vi "HEWH RLT Channel Test Labels.vi"(0 "LV Program":T3=enum."HEWH", 11 "Error In":errorcluster) -> (4 "Station A":T2, 6 "Station B":T2, 8 "Station C":T2, 10 "Station D":T2, 15 "Error Out":errorcluster)   [LabVIEW 2023]
uses:
  Type Definitions/HEWH Channel Label RLT.ctl
  Custom Instrument Control/MW100/Type Definitions/Station ID Selector.ctl
  Type Definitions/HEWH RLT Stations.ctl
  Type Definitions/HEWH Label Channel.ctl
  Utility/Save File/File Setup (Public)/Type Definition/Save File DOE LabView Program.ctl
  Type Definitions/HEWH Agilent Cluster.ctl
  Custom Instrument Control/MW100/Type Definitions/HEWH MW100 Channel Numbers.ctl
  Type Definitions/PRAT Channel Settings.ctl
  <vilib>/Utility/file.llb/Write Delimited Spreadsheet (string).vi
  <vilib>/Utility/file.llb/Read Delimited Spreadsheet (string).vi
  Utility/Save File/File Setup.lvlib
panel:
  out "Agilent Labels_Channels":T1[](array[typedef])
  in  "Tab Control":enum32{"Data Output", "Error"}(tab)
  out "Raw Data (Read)":string[][](array[string])
  out "Description":string="Thermocouple Setup"
  in  "Read":bool
  in  "Write":bool
  in  "Initialize":bool
  in  "Complete":bool
  in  "Panel 3":T4[][](array[typedef])=[[{"Label"="T3-1", "Unit"=enum.""}, {"Label"="T3-2", "Unit"=enum.""}, {"Label"="T3-3", "Unit"=enum.""}, {"Label"="T3-4", "Unit"=enum.""}, {"Label"="T3-5", "Unit"=enum.""}, {"Label"="T3-6", "Unit"=enum.""}], [{"Label"="T3-7", "Unit"=enum.""}, {"Label"="T3-8", "Unit"=enum.""}, {"Label"="T3-9", "Unit"=enum.""}, {"Label"="T3-10", "Unit"=enum.""}, {"Label"="T3-11", "Unit"=enum.""}, {"Label"="T3-12", "Unit"=enum.""}], [{"Label"="T3-13", "Unit"=enum.""}, {"Label"="T3-14", "Unit"=enum.""}, {"Label"="T3-15", "Unit"=enum.""}, {"Label"="T3-16", "Unit"=enum.""}, {"Label"="T3-17", "Unit"=enum.""}, {"Label"="T3-18", "Unit"=enum.""}]]
  in  "Panel 2":T4[][](array[typedef])=[[{"Label"="T2-1", "Unit"=enum.""}, {"Label"="T2-2", "Unit"=enum.""}, {"Label"="T2-3", "Unit"=enum.""}, {"Label"="T2-4", "Unit"=enum.""}, {"Label"="T2-5", "Unit"=enum.""}, {"Label"="T2-6", "Unit"=enum.""}], [{"Label"="T2-7", "Unit"=enum.""}, {"Label"="T2-8", "Unit"=enum.""}, {"Label"="T2-9", "Unit"=enum.""}, {"Label"="T2-10", "Unit"=enum.""}, {"Label"="T2-11", "Unit"=enum.""}, {"Label"="T2-12", "Unit"=enum.""}], [{"Label"="T2-13", "Unit"=enum.""}, {"Label"="T2-14", "Unit"=enum.""}, {"Label"="T2-15", "Unit"=enum.""}, {"Label"="T2-16", "Unit"=enum.""}, {"Label"="T2-17", "Unit"=enum.""}, {"Label"="T2-18", "Unit"=enum.""}]]
  in  "Panel 1":T4[][](array[typedef])=[[{"Label"="T1 - IN", "Unit"=enum."A"}, {"Label"="T1 - OUT", "Unit"=enum."A"}, {"Label"="T2 - IN", "Unit"=enum."B"}, {"Label"="T2 - OUT", "Unit"=enum."B"}, {"Label"="T3 - IN", "Unit"=enum."C"}, {"Label"="T3 - OUT", "Unit"=enum."C"}], [{"Label"="T4 - IN", "Unit"=enum."D"}, {"Label"="T4 - OUT", "Unit"=enum."D"}, {"Label"="T1-9", "Unit"=enum.""}, {"Label"="T1-10", "Unit"=enum.""}, {"Label"="T1-11", "Unit"=enum.""}, {"Label"="T1-12", "Unit"=enum.""}], [{"Label"="T1-13", "Unit"=enum.""}, {"Label"="T1-14", "Unit"=enum.""}, {"Label"="T1-15", "Unit"=enum.""}, {"Label"="T1-16", "Unit"=enum.""}, {"Label"="T1-17", "Unit"=enum.""}, {"Label"="T1-18", "Unit"=enum.""}]]
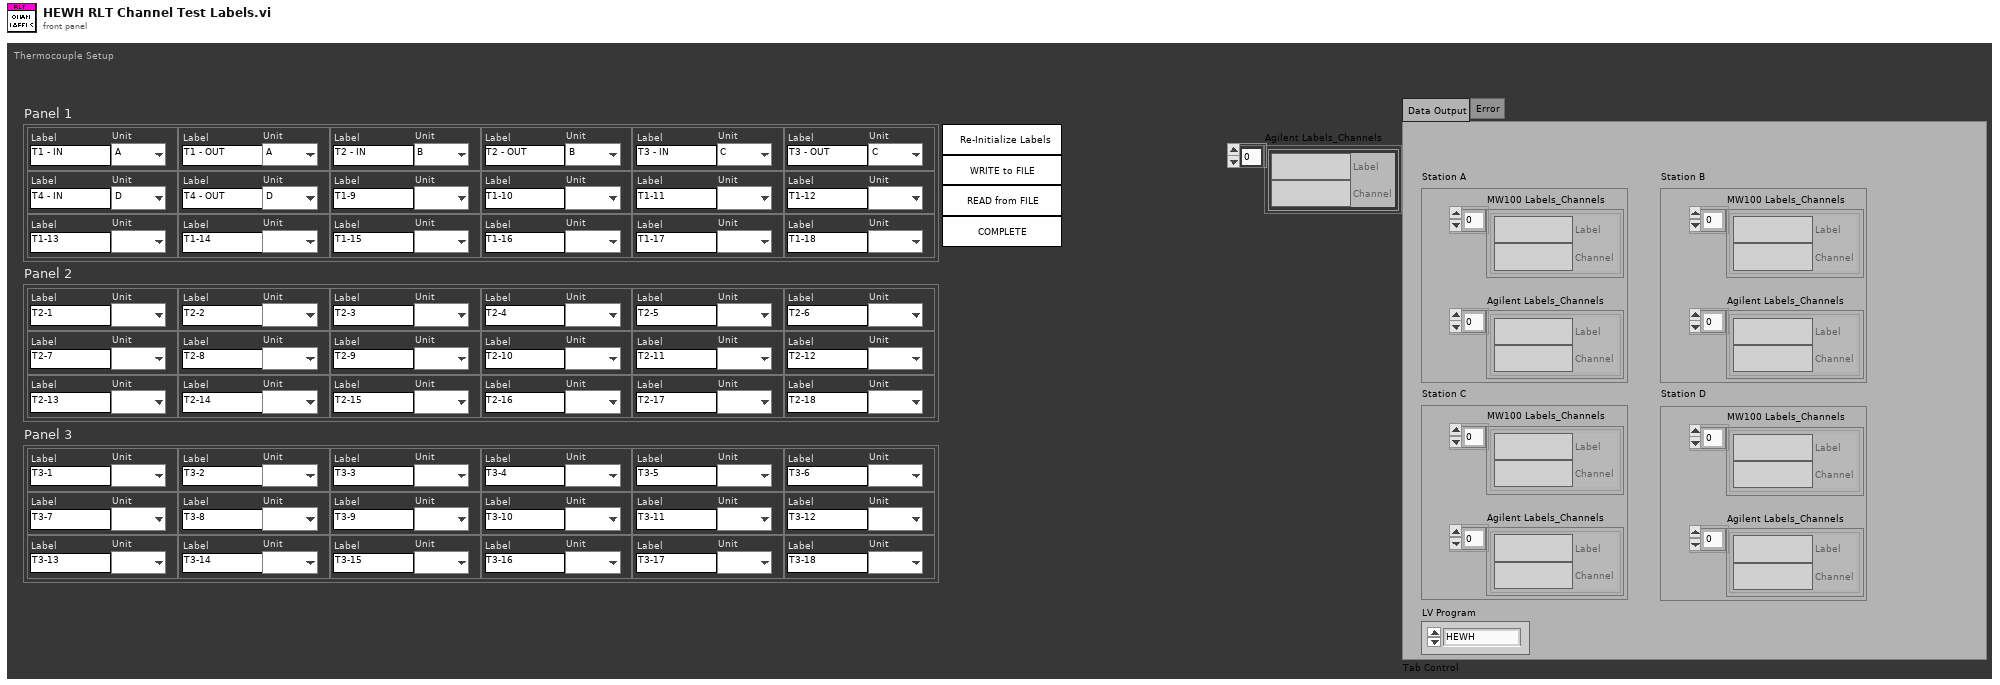
[diagram p1: front panel]
types:
  T1 = typedef "HEWH Label Channel.ctl" = cluster{"Label":string, "Channel":string}
  T2 = typedef "HEWH RLT Stations.ctl" = cluster{"MW100 Labels_Channels":T1[], "Agilent Labels_Channels":T1[]}
  T3 = typedef "File Setup.lvlib/Save File DOE LabView Program.ctl" = enum16{"No Name Found", "DOE Stand", "Dishwasher Kitchen", "Portable Stand", "HEWH", "Dryer", "Dryer WILT", "HCC", "PRAT", "HEWH RLT", "Refrigeration", "Gas Water Heater"}
  T4 = typedef "HEWH Channel Label RLT.ctl" = cluster{"Label":string, "Unit":T5}
  T5 = typedef "Station ID Selector.ctl" = enum16{"", "A", "B", "C", "D", "Global"}
  T6 = typedef "HEWH Agilent Cluster.ctl" = cluster{"Label":string, "Agilent Channel":string, "Panel ID":string, "Source":string, "Temperature":dbl}
  T7 = enum8{"Enabled", "Disabled", "Disabled and Grayed Out"}
  T8 = typedef "PRAT Channel Settings.ctl" = string
  T9 = typedef "HEWH MW100 Channel Numbers.ctl" = string
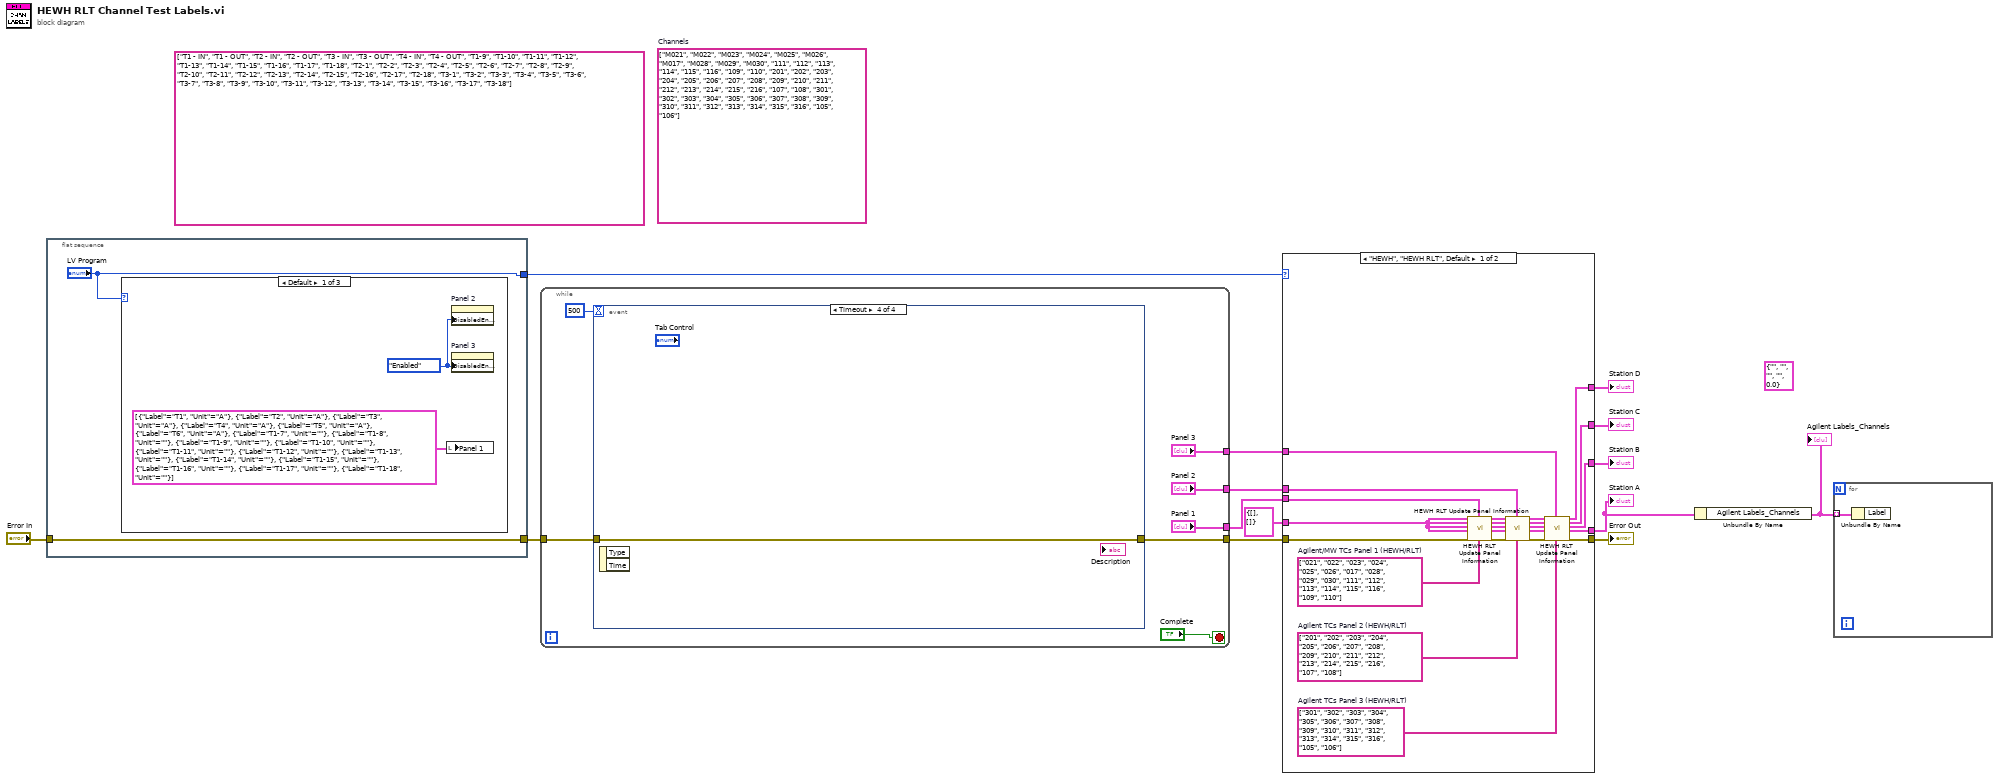
[diagram p0: block diagram]
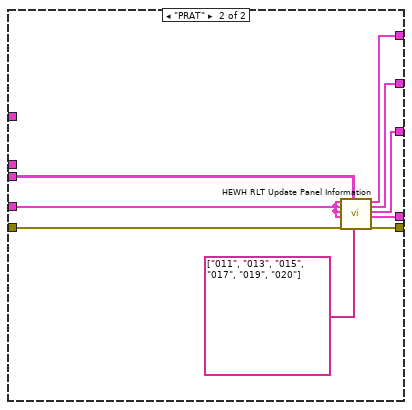
[diagram p2: hidden frame]
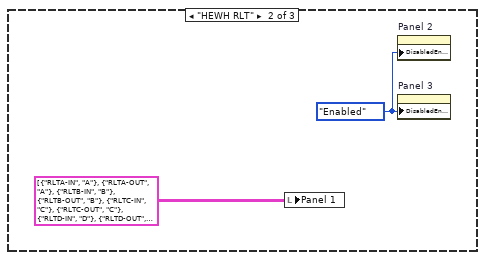
[diagram p3: hidden frame]
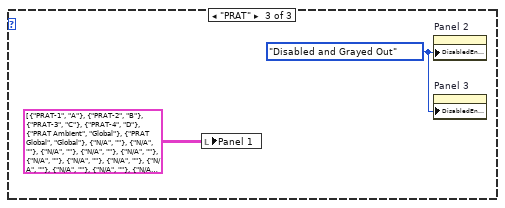
[diagram p4: hidden frame]
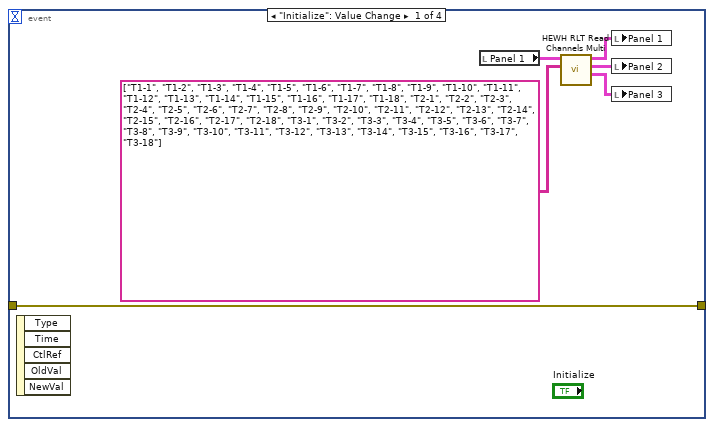
[diagram p5: hidden frame]
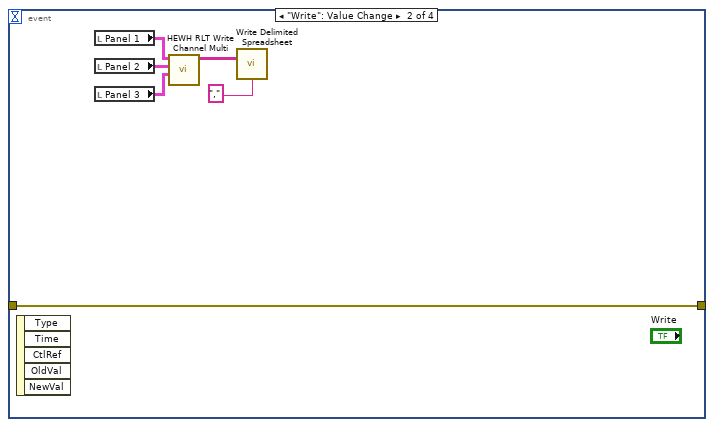
[diagram p6: hidden frame]
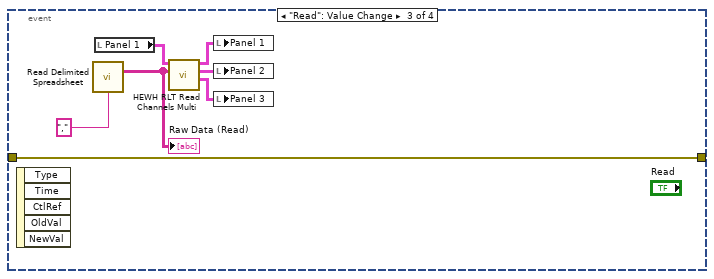
[diagram p7: hidden frame]
diagram:
  (unwired) T6 {"Label"="", "Agilent Channel"="", "Panel ID"="", "Source"="", "Temperature"=0.0} ("Agilent Cluster")
  (unwired) string[][] [["M021", "M022", "M023", "M024", "M025", "M026"], ["M017", "M028", "M029", "M030", "111", "112"], ["113", "114", "115", "116", "109", "110"], ["201", "202", "203", "204", "205", "206"], ["207", "208", "209", "210", "211", "212"], ["213", "214", "215", "216", "107", "108"], ["301", "302", "303", "304", "305", "306"], ["307", "308", "309", "310", "311", "312"], ["313", "314", "315", "316", "105", "106"]]  # Channels
  (unwired) string[][] [["T1 - IN", "T1 - OUT", "T2 - IN", "T2 - OUT", "T3 - IN", "T3 - OUT"], ["T4 - IN", "T4 - OUT", "T1-9", "T1-10", "T1-11", "T1-12"], ["T1-13", "T1-14", "T1-15", "T1-16", "T1-17", "T1-18"], ["T2-1", "T2-2", "T2-3", "T2-4", "T2-5", "T2-6"], ["T2-7", "T2-8", "T2-9", "T2-10", "T2-11", "T2-12"], ["T2-13", "T2-14", "T2-15", "T2-16", "T2-17", "T2-18"], ["T3-1", "T3-2", "T3-3", "T3-4", "T3-5", "T3-6"], ["T3-7", "T3-8", "T3-9", "T3-10", "T3-11", "T3-12"], ["T3-13", "T3-14", "T3-15", "T3-16", "T3-17", "T3-18"]] ("Array")
  n1 = flat-sequence {
    tunnel: "Error In" -> [w16]
    tunnel: [w16] -> w5
    tunnel: ["LV Program"] -> w3
    frame #0 {
      n2 = case shown="Default" "LV Program" {
        frame Default {
          w18 = T7."Enabled" ("Disabled")
          n3 = local write "Panel 1"(T4[][] [[{"Label"="T1", "Unit"=enum."A"}, {"Label"="T2", "Unit"=enum."A"}, {"Label"="T3", "Unit"=enum."A"}, {"Label"="T4", "Unit"=enum."A"}, {"Label"="T5", "Unit"=enum."A"}, {"Label"="T6", "Unit"=enum."A"}], [{"Label"="T1-7", "Unit"=enum.""}, {"Label"="T1-8", "Unit"=enum.""}, {"Label"="T1-9", "Unit"=enum.""}, {"Label"="T1-10", "Unit"=enum.""}, {"Label"="T1-11", "Unit"=enum.""}, {"Label"="T1-12", "Unit"=enum.""}], [{"Label"="T1-13", "Unit"=enum.""}, {"Label"="T1-14", "Unit"=enum.""}, {"Label"="T1-15", "Unit"=enum.""}, {"Label"="T1-16", "Unit"=enum.""}, {"Label"="T1-17", "Unit"=enum.""}, {"Label"="T1-18", "Unit"=enum.""}]] ("Panel 1")) -> ()
          n4 = property on="Panel 2" class="Arr (strict)"("DisabledEnum"=w18) -> ()  [unwired: 2 in, 2 out]
          n5 = property on="Panel 3" class="Arr (strict)"("DisabledEnum"=w18) -> ()  [unwired: 2 in, 2 out]
        }
        frame "HEWH RLT" {
          w20 = T7."Enabled" ("Disabled")
          n6 = local write "Panel 1"(T4[][] [[{"Label"="RLTA-IN", "Unit"=enum."A"}, {"Label"="RLTA-OUT", "Unit"=enum."A"}, {"Label"="RLTB-IN", "Unit"=enum."B"}, {"Label"="RLTB-OUT", "Unit"=enum."B"}, {"Label"="RLTC-IN", "Unit"=enum."C"}, {"Label"="RLTC-OUT", "Unit"=enum."C"}], [{"Label"="RLTD-IN", "Unit"=enum."D"}, {"Label"="RLTD-OUT", "Unit"=enum."D"}, {"Label"="T1-9", "Unit"=enum.""}, {"Label"="T1-10", "Unit"=enum.""}, {"Label"="T1-11", "Unit"=enum.""}, {"Label"="T1-12", "Unit"=enum.""}], [{"Label"="T1-13", "Unit"=enum.""}, {"Label"="T1-14", "Unit"=enum.""}, {"Label"="T1-15", "Unit"=enum.""}, {"Label"="T1-16", "Unit"=enum.""}, {"Label"="T1-17", "Unit"=enum.""}, {"Label"="T1-18", "Unit"=enum.""}]] ("Panel 1")) -> ()
          n7 = property on="Panel 2" class="Arr (strict)"("DisabledEnum"=w20) -> ()  [unwired: 2 in, 2 out]
          n8 = property on="Panel 3" class="Arr (strict)"("DisabledEnum"=w20) -> ()  [unwired: 2 in, 2 out]
        }
        frame "PRAT" {
          w22 = T7."Disabled and Grayed Out" ("Disabled")
          n9 = local write "Panel 1"(T4[][] [[{"Label"="PRAT-1", "Unit"=enum."A"}, {"Label"="PRAT-2", "Unit"=enum."B"}, {"Label"="PRAT-3", "Unit"=enum."C"}, {"Label"="PRAT-4", "Unit"=enum."D"}, {"Label"="PRAT Ambient", "Unit"=enum."Global"}, {"Label"="PRAT Global", "Unit"=enum."Global"}], [{"Label"="N/A", "Unit"=enum.""}, {"Label"="N/A", "Unit"=enum.""}, {"Label"="N/A", "Unit"=enum.""}, {"Label"="N/A", "Unit"=enum.""}, {"Label"="N/A", "Unit"=enum.""}, {"Label"="N/A", "Unit"=enum.""}], [{"Label"="N/A", "Unit"=enum.""}, {"Label"="N/A", "Unit"=enum.""}, {"Label"="N/A", "Unit"=enum.""}, {"Label"="N/A", "Unit"=enum.""}, {"Label"="N/A", "Unit"=enum.""}, {"Label"="N/A", "Unit"=enum.""}]] ("Panel 1")) -> ()
          n10 = property on="Panel 2" class="Arr (strict)"("DisabledEnum"=w22) -> ()  [unwired: 2 in, 2 out]
          n11 = property on="Panel 3" class="Arr (strict)"("DisabledEnum"=w22) -> ()  [unwired: 2 in, 2 out]
        }
      }
    }
  }
  n12 = while {
    tunnel: ["Panel 1"] -> w9
    tunnel: ["Panel 2"] -> w8
    tunnel: ["Panel 3"] -> w7
    tunnel: w5 -> [w24]
    tunnel: [w23] -> w10
    stop <- "Complete" stop-if-true
    n13 = event shown="[3] Timeout" {
      selector: _ -> [_ _ _ _]
      dyn-events: _ -> [_ _ _ _]
      timeout: 500 -> [_ _ _ _]
      tunnel: w24 -> [w30 w37 w43 w49]
      tunnel: [w30 w37 w43 w49] -> w23
      event "Initialize": Value Change {
        n14 = event-data() -> ()  [unwired: 1 in, 5 out]
        n15 = local read "Panel 1"() -> (w34:T4[][])
        n16 = call "HEWH RLT Read Channels Multi.vi"("Raw Data Input"=string[][] [["T1-1", "T1-2", "T1-3", "T1-4", "T1-5", "T1-6"], ["T1-7", "T1-8", "T1-9", "T1-10", "T1-11", "T1-12"], ["T1-13", "T1-14", "T1-15", "T1-16", "T1-17", "T1-18"], ["T2-1", "T2-2", "T2-3", "T2-4", "T2-5", "T2-6"], ["T2-7", "T2-8", "T2-9", "T2-10", "T2-11", "T2-12"], ["T2-13", "T2-14", "T2-15", "T2-16", "T2-17", "T2-18"], ["T3-1", "T3-2", "T3-3", "T3-4", "T3-5", "T3-6"], ["T3-7", "T3-8", "T3-9", "T3-10", "T3-11", "T3-12"], ["T3-13", "T3-14", "T3-15", "T3-16", "T3-17", "T3-18"]] ("Array"), "Panel Input"=w34) -> ("Panel 3"=w31:T4[][], "Panel 2"=w32:T4[][], "Panel 1"=w33:T4[][])  [unwired: 6 in, 1 out]
        n17 = local write "Panel 1"(w33) -> ()
        n18 = local write "Panel 2"(w32) -> ()
        n19 = local write "Panel 3"(w31) -> ()
      }
      event "Write": Value Change {
        n20 = event-data() -> ()  [unwired: 1 in, 5 out]
        n21 = local read "Panel 1"() -> (w41:T4[][])
        n22 = local read "Panel 2"() -> (w39:T4[][])
        n23 = local read "Panel 3"() -> (w38:T4[][])
        n24 = call "HEWH RLT Write Channel Multi.vi"("Panel 3"=w38, "Panel 2"=w39, "Panel 1"=w41) -> ("Write Array Out"=w36:string[][])  [unwired: 7 in, 1 out]
        n25 = call-poly <vilib>:"Write Delimited Spreadsheet.vi"("2D data"=w36, "delimiter (\\t)"="," ("delimiter (\\t)")) -> ()  [unwired: 12 in, 2 out]
      }
      event "Read": Value Change {
        n26 = event-data() -> ()  [unwired: 1 in, 5 out]
        n27 = call-poly <vilib>:"Read Delimited Spreadsheet.vi"("delimiter (\\t)"="," ("delimiter (\\t)")) -> ("all rows"=w42:string[][])  [unwired: 9 in, 5 out]
        "Raw Data (Read)" <- w42
        n28 = local read "Panel 1"() -> (w47:T4[][])
        n29 = call "HEWH RLT Read Channels Multi.vi"("Raw Data Input"=w42, "Panel Input"=w47) -> ("Panel 3"=w44:T4[][], "Panel 2"=w45:T4[][], "Panel 1"=w46:T4[][])  [unwired: 6 in, 1 out]
        n30 = local write "Panel 1"(w46) -> ()
        n31 = local write "Panel 2"(w45) -> ()
        n32 = local write "Panel 3"(w44) -> ()
      }
      event Timeout {
        n33 = event-data() -> ()  [unwired: 1 in, 2 out]
      }
    }
  }
  n34 = case shown="\"HEWH\", \"HEWH RLT\", Default" w3 {
    tunnel: [w61 w78] -> w14
    tunnel: [w60 w77] -> w13
    tunnel: [w59 w76] -> w12
    tunnel: [w58 w75] -> w2
    tunnel: [w55 w74] -> w11
    tunnel: w10 -> [w54 w79]
    tunnel: w9 -> [w53 w81]
    tunnel: w8 -> [w52 _]
    tunnel: w7 -> [w51 _]
    tunnel: T2 {"MW100 Labels_Channels"=[], "Agilent Labels_Channels"=[]} ("Station A") -> [w50 w80]
    frame "HEWH", "HEWH RLT", Default {
      w62 = T9[] ["301", "302", "303", "304", "305", "306", "307", "308", "309", "310", "311", "312", "313", "314", "315", "316", "105", "106"]  # Agilent TCs Panel 3 (HEWH/RLT)
      w63 = T9[] ["201", "202", "203", "204", "205", "206", "207", "208", "209", "210", "211", "212", "213", "214", "215", "216", "107", "108"]  # Agilent TCs Panel 2 (HEWH/RLT)
      w72 = T9[] ["021", "022", "023", "024", "025", "026", "017", "028", "029", "030", "111", "112", "113", "114", "115", "116", "109", "110"]  # Agilent/MW TCs Panel 1 (HEWH/RLT)
      n35 = call "HEWH RLT Update Panel Information.vi"("Station D In"=w50, "Station C In"=w50, "Station B In"=w50, "Station A In"=w50, "Error In"=w54, "Panel"=w53, "MW 100 Channel Input"=w72) -> ("Station D Out"=w71:T2, "Station C Out"=w70:T2, "Station B Out"=w69:T2, "Station A Out"=w68:T2, "Error Out"=w57:errorcluster)  [unwired: 8 in]
      n36 = call "HEWH RLT Update Panel Information.vi"("Station D In"=w71, "Station C In"=w70, "Station B In"=w69, "Station A In"=w68, "Error In"=w57, "Panel"=w52, "MW 100 Channel Input"=w63) -> ("Station D Out"=w67:T2, "Station C Out"=w66:T2, "Station B Out"=w65:T2, "Station A Out"=w64:T2, "Error Out"=w56:errorcluster)  [unwired: 8 in]
      n37 = call "HEWH RLT Update Panel Information.vi"("Station D In"=w67, "Station C In"=w66, "Station B In"=w65, "Station A In"=w64, "Error In"=w56, "Panel"=w51, "MW 100 Channel Input"=w62) -> ("Station D Out"=w61:T2, "Station C Out"=w60:T2, "Station B Out"=w59:T2, "Station A Out"=w58:T2, "Error Out"=w55:errorcluster)  [unwired: 8 in]
    }
    frame "PRAT" {
      n38 = call "HEWH RLT Update Panel Information.vi"("Station D In"=w80, "Station C In"=w80, "Station B In"=w80, "Station A In"=w80, "Error In"=w79, "Panel"=w81, "MW 100 Channel Input"=T8[] ["011", "013", "015", "017", "019", "020"]) -> ("Station D Out"=w78:T2, "Station C Out"=w77:T2, "Station B Out"=w76:T2, "Station A Out"=w75:T2, "Error Out"=w74:errorcluster)  [unwired: 8 in]
    }
  }
  "Station C" <- w13
  "Station A" <- w2
  "Station B" <- w12
  "Station D" <- w14
  "Error Out" <- w11
  n39 = Unbundle By Name(w2) -> ("Agilent Labels_Channels"=w1:T1[])
  "Agilent Labels_Channels" <- w1
  n40 = for {
    tunnel: w1 -> [w82] mode=indexing
    n41 = Unbundle By Name(w82) -> ()  [unwired: 1 out]
  }
